vi "GeoData.vi"() -> ()   [LabVIEW 2017] (continued)
Hope\tIN\tBartholomew County\tH1\n47234\t18005\tFlat rock\tIN\tBartholomew County\tH1\n47244\t18005\tHartsville\tIN\tBartholomew County\tH1\n47226\t18005\tClifford\tIN\tBartholomew County\tH1\n47944\t18007\tFowler\tIN\tBenton County\tH1\n47917\t18007\tAmbia\tIN\tBenton County\tH1\n47975\t18007\tPine village\tIN\tBenton County\tH1\n47986\t18007\tTempleton\tIN\tBenton County\tH1\n47971\t18007\tOxford\tIN\tBenton County\tH1\n47948\t18007\tGoodland\tIN\tBenton County\tH1\n47970\t18007\tOtterbein\tIN\tBenton County\tH1\n47942\t18007\tEarl park\tIN\tBenton County\tH1\n47921\t18007\tBoswell\tIN\tBenton County\tH1\n47977\t18007\tRemington\tIN\tBenton County\tH1\n47995\t18007\tWolcott\tIN\tBenton County\tH1\n47359\t18009\tMontpelier\tIN\tBlackford County\tH1\n47348\t18009\tHartford city\tIN\tBlackford County\tH1\n47303\t18009\tMuncie\tIN\tBlackford County\tH1\n47338\t18009\tEaton\tIN\tBlackford County\tH1\n46952\t18009\tMarion\tIN\tBlackford County\tH1\n46989\t18009\tUpland\tIN\tBlackford County\tH1\n47336\t18009\tDunkirk\tIN\tBlackford County\tH1\n47369\t18009\tPennville\tIN\tBlackford County\tH1\n46147\t18011\tJamestown\tIN\tBoone County\tH1\n46268\t18011\tIndianapolis\tIN\tBoone County\tH1\n46102\t18011\tAdvance\tIN\tBoone County\tH1\n46041\t18011\tFrankfort\tIN\tBoone County\tH1\n46069\t18011\tSheridan\tIN\tBoone County\tH1\n46035\t18011\tColfax\tIN\tBoone County\tH1\n46112\t18011\tBrownsburg\tIN\tBoone County\tH1\n46052\t18011\tLebanon\tIN\tBoone County\tH1\n46077\t18011\tZionsville\tIN\tBoone County\tH1\n46278\t18011\tIndianapolis\tIN\tBoone County\tH1\n46032\t18011\tCarmel\tIN\tBoone County\tH1\n47933\t18011\tCrawfordsville\tIN\tBoone County\tH1\n47968\t18011\tNew ross\tIN\tBoone County\tH1\n46075\t18011\tWhitestown\tIN\tBoone County\tH1\n46167\t18011\tPittsboro\tIN\tBoone County\tH1\n46050\t18011\tKirklin\tIN\tBoone County\tH1\n46149\t18011\tLizton\tIN\tBoone County\tH1\n46071\t18011\tThorntown\tIN\tBoone County\tH1\n47274\t18013\tSeymour\tIN\tBrown County\tH1\n47448\t18013\tNashville\tIN\tBrown County\tH1\n47435\t18013\tHelmsburg\tIN\tBrown County\tH1\n46181\t18013\tTrafalgar\tIN\tBrown County\tH1\n47468\t18013\tUnionville\tIN\tBrown County\tH1\n47235\t18013\tFreetown\tIN\tBrown County\tH1\n47401\t18013\tBloomington\tIN\tBrown County\tH1\n46160\t18013\tMorgantown\tIN\tBrown County\tH1\n46164\t18013\tNineveh\tIN\tBrown County\tH1\n47201\t18013\tColumbus\tIN\tBrown County\tH1\n46915\t18015\tBurlington\tIN\tCarroll County\tH1\n47950\t18015\tIdaville\tIN\tCarroll County\tH1\n46929\t18015\tFlora\tIN\tCarroll County\tH1\n46917\t18015\tCamden\tIN\tCarroll County\tH1\n46913\t18015\tBringhurst\tIN\tCarroll County\tH1\n46041\t18015\tFrankfort\tIN\tCarroll County\tH1\n47960\t18015\tMonticello\tIN\tCarroll County\tH1\n46916\t18015\tBurrows\tIN\tCarroll County\tH1\n47926\t18015\tBurnettsville\tIN\tCarroll County\tH1\n46977\t18015\tRockfield\tIN\tCarroll County\tH1\n47997\t18015\tYeoman\tIN\tCarroll County\tH1\n46065\t18015\tRossville\tIN\tCarroll County\tH1\n46947\t18015\tLogansport\tIN\tCarroll County\tH1\n47905\t18015\tLafayette\tIN\tCarroll County\tH1\n47923\t18015\tBrookston\tIN\tCarroll County\tH1\n47920\t18015\tBattle ground\tIN\tCarroll County\tH1\n46920\t18015\tCutler\tIN\tCarroll County\tH1\n46923\t18015\tDelphi\tIN\tCarroll County\tH1\n46979\t18015\tRussiaville\tIN\tCarroll County\tH1\n46998\t18017\tYoung america\tIN\tCass County\tH1\n46917\t18017\tCamden\tIN\tCass County\tH1\n46926\t18017\tDenver\tIN\tCass County\tH1\n47926\t18017\tBurnettsville\tIN\tCass County\tH1\n46951\t18017\tMacy\tIN\tCass County\tH1\n46988\t18017\tTwelve mile\tIN\tCass County\tH1\n46978\t18017\tRoyal center\tIN\tCass County\tH1\n46947\t18017\tLogansport\tIN\tCass County\tH1\n46932\t18017\tGalveston\tIN\tCass County\tH1\n46950\t18017\tLucerne\tIN\tCass County\tH1\n46961\t18017\tNew waverly\tIN\tCass County\tH1\n46967\t18017\tOnward\tIN\tCass County\tH1\n46901\t18017\tKokomo\tIN\tCass County\tH1\n46970\t18017\tPeru\tIN\tCass County\tH1\n46994\t18017\tWalton\tIN\tCass County\tH1\n46942\t18017\tLake cicott\tIN\tCass County\tH1\n47119\t18019\tFloyds knobs\tIN\tClark County\tH1\n47141\t18019\tMarysville\tIN\tClark County\tH1\n47163\t18019\tOtisco\tIN\tClark County\tH1\n47243\t18019\tHanover\tIN\tClark County\tH1\n47130\t18019\tJeffersonville\tIN\tClark County\tH1\n47165\t18019\tPekin\tIN\tClark County\tH1\n47147\t18019\tNabb\tIN\tClark County\tH1\n47111\t18019\tCharlestown\tIN\tClark County\tH1\n47131\t18019\tJeffersonville\tIN\tClark County\tH1\n47172\t18019\tSellersburg\tIN\tClark County\tH1\n47190\t18019\tJeffersonville\tIN\tClark County\tH1\n47150\t18019\tNew albany\tIN\tClark County\tH1\n47126\t18019\tHenryville\tIN\tClark County\tH1\n47162\t18019\tNew washington\tIN\tClark County\tH1\n47106\t18019\tBorden\tIN\tClark County\tH1\n47143\t18019\tMemphis\tIN\tClark County\tH1\n47104\t18019\tBethlehem\tIN\tClark County\tH1\n47129\t18019\tClarksville\tIN\tClark County\tH1\n47138\t18019\tLexington\tIN\tClark County\tH1\n47177\t18019\tUnderwood\tIN\tClark County\tH1\n47802\t18021\tTerre haute\tIN\tClay County\tH1\n47840\t18021\tCenterpoint\tIN\tClay County\tH1\n47845\t18021\tCoalmont\tIN\tClay County\tH1\n47853\t18021\tHarmony\tIN\tClay County\tH1\n47857\t18021\tKnightsville\tIN\tClay County\tH1\n47868\t18021\tPoland\tIN\tClay County\tH1\n47427\t18021\tCoal city\tIN\tClay County\tH1\n47858\t18021\tLewis\tIN\tClay County\tH1\n47841\t18021\tClay city\tIN\tClay County\tH1\n47881\t18021\tStaunton\tIN\tClay County\tH1\n47834\t18021\tBrazil\tIN\tClay County\tH1\n47879\t18021\tShelburn\tIN\tClay County\tH1\n47803\t18021\tTerre haute\tIN\tClay County\tH1\n47438\t18021\tJasonville\tIN\tClay County\tH1\n47874\t18021\tRosedale\tIN\tClay County\tH1\n47846\t18021\tCory\tIN\tClay County\tH1\n47837\t18021\tCarbon\tIN\tClay County\tH1\n47833\t18021\tBowling green\tIN\tClay County\tH1\n46039\t18023\tForest\tIN\tClinton County\tH1\n46041\t18023\tFrankfort\tIN\tClinton County\tH1\n46069\t18023\tSheridan\tIN\tClinton County\tH1\n46035\t18023\tColfax\tIN\tClinton County\tH1\n46067\t18023\tSedalia\tIN\tClinton County\tH1\n46065\t18023\tRossville\tIN\tClinton County\tH1\n46057\t18023\tMichigantown\tIN\tClinton County\tH1\n46049\t18023\tKempton\tIN\tClinton County\tH1\n46058\t18023\tMulberry\tIN\tClinton County\tH1\n46050\t18023\tKirklin\tIN\tClinton County\tH1\n46979\t18023\tRussiaville\tIN\tClinton County\tH1\n46071\t18023\tThorntown\tIN\tClinton County\tH1\n47930\t18023\tClarks hill\tIN\tClinton County\tH1\n47175\t18025\tTaswell\tIN\tCrawford County\tH1\n47576\t18025\tSaint croix\tIN\tCrawford County\tH1\n47116\t18025\tEckerty\tIN\tCrawford County\tH1\n47123\t18025\tGrantsburg\tIN\tCrawford County\tH1\n47174\t18025\tSulphur\tIN\tCrawford County\tH1\n47145\t18025\tMilltown\tIN\tCrawford County\tH1\n47140\t18025\tMarengo\tIN\tCrawford County\tH1\n47112\t18025\tCorydon\tIN\tCrawford County\tH1\n47137\t18025\tLeavenworth\tIN\tCrawford County\tH1\n47118\t18025\tEnglish\tIN\tCrawford County\tH1\n47513\t18025\tBirdseye\tIN\tCrawford County\tH1\n47553\t18027\tLoogootee\tIN\tDaviess County\tH1\n47562\t18027\tOdon\tIN\tDaviess County\tH1\n47529\t18027\tElnora\tIN\tDaviess County\tH1\n47501\t18027\tWashington\tIN\tDaviess County\tH1\n47519\t18027\tCannelburg\tIN\tDaviess County\tH1\n47568\t18027\tPlainville\tIN\tDaviess County\tH1\n47558\t18027\tMontgomery\tIN\tDaviess County\tH1\n47449\t18027\tNewberry\tIN\tDaviess County\tH1\n47001\t18029\tAurora\tIN\tDearborn County\tH1\n47018\t18029\tDillsboro\tIN\tDearborn County\tH1\n47060\t18029\tWest harrison\tIN\tDearborn County\tH1\n47012\t18029\tBrookville\tIN\tDearborn County\tH1\n47032\t18029\tMoores hill\tIN\tDearborn County\tH1\n47025\t18029\tLawrenceburg\tIN\tDearborn County\tH1\n47022\t18029\tGuilford\tIN\tDearborn County\tH1\n47041\t18029\tSunman\tIN\tDearborn County\tH1\n47031\t18029\tMilan\tIN\tDearborn County\tH1\n46156\t18031\tMilroy\tIN\tDecatur County\tH1\n47240\t18031\tGreensburg\tIN\tDecatur County\tH1\n47225\t18031\tClarksburg\tIN\tDecatur County\tH1\n47263\t18031\tNew point\tIN\tDecatur County\tH1\n46173\t18031\tRushville\tIN\tDecatur County\tH1\n47272\t18031\tSaint paul\tIN\tDecatur County\tH1\n47283\t18031\tWestport\tIN\tDecatur County\tH1\n47006\t18031\tBatesville\tIN\tDecatur County\tH1\n47246\t18031\tHope\tIN\tDecatur County\tH1\n47244\t18031\tHartsville\tIN\tDecatur County\tH1\n46747\t18033\tHudson\tIN\tDeKalb County\tH1\n46742\t18033\tHamilton\tIN\tDeKalb County\tH1\n46730\t18033\tCorunna\tIN\tDeKalb County\tH1\n46748\t18033\tHuntertown\tIN\tDeKalb County\tH1\n46743\t18033\tHarlan\tIN\tDeKalb County\tH1\n46755\t18033\tKendallville\tIN\tDeKalb County\tH1\n46793\t18033\tWaterloo\tIN\tDeKalb County\tH1\n46706\t18033\tAuburn\tIN\tDeKalb County\tH1\n46710\t18033\tAvilla\tIN\tDeKalb County\tH1\n46785\t18033\tSaint joe\tIN\tDeKalb County\tH1\n46738\t18033\tGarrett\tIN\tDeKalb County\tH1\n46763\t18033\tLaotto\tIN\tDeKalb County\tH1\n46721\t18033\tButler\tIN\tDeKalb County\tH1\n46705\t18033\tAshley\tIN\tDeKalb County\tH1\n46788\t18033\tSpencerville\tIN\tDeKalb County\tH1\n46012\t18035\tAnderson\tIN\tDelaware County\tH1\n47306\t18035\tMuncie\tIN\tDelaware County\tH1\n47302\t18035\tMuncie\tIN\tDelaware County\tH1\n47320\t18035\tAlbany\tIN\tDelaware County\tH1\n47386\t18035\tSpringport\tIN\tDelaware County\tH1\n47303\t18035\tMuncie\tIN\tDelaware County\tH1\n47338\t18035\tEaton\tIN\tDelaware County\tH1\n47342\t18035\tGaston\tIN\tDelaware County\tH1\n47304\t18035\tMuncie\tIN\tDelaware County\tH1\n47396\t18035\tYorktown\tIN\tDelaware County\tH1\n47308\t18035\tMuncie\tIN\tDelaware County\tH1\n47383\t18035\tSelma\tIN\tDelaware County\tH1\n46001\t18035\tAlexandria\tIN\tDelaware County\tH1\n47336\t18035\tDunkirk\tIN\tDelaware County\tH1\n47307\t18035\tMuncie\tIN\tDelaware County\tH1\n47367\t18035\tOakville\tIN\tDelaware County\tH1\n46017\t18035\tAnderson\tIN\tDelaware County\tH1\n46070\t18035\tSummitville\tIN\tDelaware County\tH1\n47356\t18035\tMiddletown\tIN\tDelaware County\tH1\n47334\t18035\tDaleville\tIN\tDelaware County\tH1\n47368\t18035\tParker city\tIN\tDelaware County\tH1\n47354\t18035\tLosantville\tIN\tDelaware County\tH1\n47305\t18035\tMuncie\tIN\tDelaware County\tH1\n47523\t18037\tDale\tIN\tDubois County\tH1\n47542\t18037\tHuntingburg\tIN\tDubois County\tH1\n47547\t18037\tJasper\tIN\tDubois County\tH1\n47575\t18037\tSaint anthony\tIN\tDubois County\tH1\n47527\t18037\tDubois\tIN\tDubois County\tH1\n47564\t18037\tOtwell\tIN\tDubois County\tH1\n47580\t18037\tSchnellville\tIN\tDubois County\tH1\n47541\t18037\tHolland\tIN\tDubois County\tH1\n47590\t18037\tVelpen\tIN\tDubois County\tH1\n47546\t18037\tJasper\tIN\tDubois County\tH1\n47432\t18037\tFrench lick\tIN\tDubois County\tH1\n47521\t18037\tCelestine\tIN\tDubois County\tH1\n47545\t18037\tIreland\tIN\tDubois County\tH1\n47532\t18037\tFerdinand\tIN\tDubois County\tH1\n47513\t18037\tBirdseye\tIN\tDubois County\tH1\n46514\t18039\tElkhart\tIN\tElkhart County\tH1\n46516\t18039\tElkhart\tIN\tElkhart County\tH1\n46567\t18039\tSyracuse\tIN\tElkhart County\tH1\n46542\t18039\tMilford\tIN\tElkhart County\tH1\n46561\t18039\tOsceola\tIN\tElkhart County\tH1\n46565\t18039\tShipshewana\tIN\tElkhart County\tH1\n46550\t18039\tNappanee\tIN\tElkhart County\tH1\n46527\t18039\tGoshen\tIN\tElkhart County\tH1\n46553\t18039\tNew paris\tIN\tElkhart County\tH1\n46517\t18039\tElkhart\tIN\tElkhart County\tH1\n46530\t18039\tGranger\tIN\tElkhart County\tH1\n46515\t18039\tElkhart\tIN\tElkhart County\tH1\n46573\t18039\tWakarusa\tIN\tElkhart County\tH1\n46526\t18039\tGoshen\tIN\tElkhart County\tH1\n46540\t18039\tMiddlebury\tIN\tElkhart County\tH1\n46528\t18039\tGoshen\tIN\tElkhart County\tH1\n46543\t18039\tMillersburg\tIN\tElkhart County\tH1\n46767\t18039\tLigonier\tIN\tElkhart County\tH1\n46507\t18039\tBristol\tIN\tElkhart County\tH1\n47331\t18041\tConnersville\tIN\tFayette County\tH1\n46127\t18041\tFalmouth\tIN\tFayette County\tH1\n47327\t18041\tCambridge city\tIN\tFayette County\tH1\n47352\t18041\tLewisville\tIN\tFayette County\tH1\n46173\t18041\tRushville\tIN\tFayette County\tH1\n46133\t18041\tGlenwood\tIN\tFayette County\tH1\n47024\t18041\tLaurel\tIN\tFayette County\tH1\n47325\t18041\tBrownsville\tIN\tFayette County\tH1\n47357\t18041\tMilton\tIN\tFayette County\tH1\n47322\t18041\tBentonville\tIN\tFayette County\tH1\n47164\t18043\tPalmyra\tIN\tFloyd County\tH1\n47119\t18043\tFloyds knobs\tIN\tFloyd County\tH1\n47165\t18043\tPekin\tIN\tFloyd County\tH1\n47172\t18043\tSellersburg\tIN\tFloyd County\tH1\n47150\t18043\tNew albany\tIN\tFloyd County\tH1\n47117\t18043\tElizabeth\tIN\tFloyd County\tH1\n47136\t18043\tLanesville\tIN\tFloyd County\tH1\n47106\t18043\tBorden\tIN\tFloyd County\tH1\n47122\t18043\tGeorgetown\tIN\tFloyd County\tH1\n47124\t18043\tGreenville\tIN\tFloyd County\tH1\n47151\t18043\tNew albany\tIN\tFloyd County\tH1\n47146\t18043\tMount saint francis\tIN\tFloyd County\tH1\n47958\t18045\tMellott\tIN\tFountain County\tH1\n47990\t18045\tWaynetown\tIN\tFountain County\tH1\n47992\t18045\tWestpoint\tIN\tFountain County\tH1\n47952\t18045\tKingman\tIN\tFountain County\tH1\n47933\t18045\tCrawfordsville\tIN\tFountain County\tH1\n47932\t18045\tCovington\tIN\tFountain County\tH1\n47987\t18045\tVeedersburg\tIN\tFountain County\tH1\n47994\t18045\tWingate\tIN\tFountain County\tH1\n47949\t18045\tHillsboro\tIN\tFountain County\tH1\n47969\t18045\tNewtown\tIN\tFountain County\tH1\n47918\t18045\tAttica\tIN\tFountain County\tH1\n47060\t18047\tWest harrison\tIN\tFranklin County\tH1\n47240\t18047\tGreensburg\tIN\tFranklin County\tH1\n47331\t18047\tConnersville\tIN\tFranklin County\tH1\n47036\t18047\tOldenburg\tIN\tFranklin County\tH1\n47010\t18047\tBath\tIN\tFranklin County\tH1\n47012\t18047\tBrookville\tIN\tFranklin County\tH1\n46173\t18047\tRushville\tIN\tFranklin County\tH1\n47353\t18047\tLiberty\tIN\tFranklin County\tH1\n47006\t18047\tBatesville\tIN\tFranklin County\tH1\n47030\t18047\tMetamora\tIN\tFranklin County\tH1\n47003\t18047\tWest college corner\tIN\tFranklin County\tH1\n47024\t18047\tLaurel\tIN\tFranklin County\tH1\n47041\t18047\tSunman\tIN\tFranklin County\tH1\n47016\t18047\tCedar grove\tIN\tFranklin County\tH1\n47035\t18047\tNew trenton\tIN\tFranklin County\tH1\n46910\t18049\tAkron\tIN\tFulton County\tH1\n46945\t18049\tLeiters ford\tIN\tFulton County\tH1\n46570\t18049\tTippecanoe\tIN\tFulton County\tH1\n46912\t18049\tAthens\tIN\tFulton County\tH1\n46951\t18049\tMacy\tIN\tFulton County\tH1\n46985\t18049\tStar city\tIN\tFulton County\tH1\n46978\t18049\tRoyal center\tIN\tFulton County\tH1\n46922\t18049\tDelong\tIN\tFulton County\tH1\n46539\t18049\tMentone\tIN\tFulton County\tH1\n46982\t18049\tSilver lake\tIN\tFulton County\tH1\n46960\t18049\tMonterey\tIN\tFulton County\tH1\n46931\t18049\tFulton\tIN\tFulton County\tH1\n46501\t18049\tArgos\tIN\tFulton County\tH1\n46950\t18049\tLucerne\tIN\tFulton County\tH1\n46511\t18049\tCulver\tIN\tFulton County\tH1\n46939\t18049\tKewanna\tIN\tFulton County\tH1\n46975\t18049\tRochester\tIN\tFulton County\tH1\n47633\t18051\tPoseyville\tIN\tGibson County\tH1\n47616\t18051\tGriffin\tIN\tGibson County\tH1\n47660\t18051\tOakland city\tIN\tGibson County\tH1\n47613\t18051\tElberfeld\tIN\tGibson County\tH1\n47665\t18051\tOwensville\tIN\tGibson County\tH1\n47648\t18051\tFort branch\tIN\tGibson County\tH1\n47666\t18051\tPatoka\tIN\tGibson County\tH1\n47725\t18051\tEvansville\tIN\tGibson County\tH1\n47654\t18051\tMackey\tIN\tGibson County\tH1\n47683\t18051\tSomerville\tIN\tGibson County\tH1\n47612\t18051\tCynthiana\tIN\tGibson County\tH1\n47639\t18051\tHaubstadt\tIN\tGibson County\tH1\n47647\t18051\tBuckskin\tIN\tGibson County\tH1\n47619\t18051\tLynnville\tIN\tGibson County\tH1\n47670\t18051\tPrinceton\tIN\tGibson County\tH1\n47640\t18051\tHazleton\tIN\tGibson County\tH1\n47649\t18051\tFrancisco\tIN\tGibson County\tH1\n46933\t18053\tGas city\tIN\tGrant County\tH1\n46930\t18053\tFowlerton\tIN\tGrant County\tH1\n46986\t18053\tSwayzee\tIN\tGrant County\tH1\n46919\t18053\tConverse\tIN\tGrant County\tH1\n46991\t18053\tVan buren\tIN\tGrant County\tH1\n46987\t18053\tSweetser\tIN\tGrant County\tH1\n47348\t18053\tHartford city\tIN\tGrant County\tH1\n47342\t18053\tGaston\tIN\tGrant County\tH1\n46957\t18053\tMatthews\tIN\tGrant County\tH1\n46952\t18053\tMarion\tIN\tGrant County\tH1\n46953\t18053\tMarion\tIN\tGrant County\tH1\n46989\t18053\tUpland\tIN\tGrant County\tH1\n46928\t18053\tFairmount\tIN\tGrant County\tH1\n46036\t18053\tElwood\tIN\tGrant County\tH1\n46938\t18053\tJonesboro\tIN\tGrant County\tH1\n46940\t18053\tLa fontaine\tIN\tGrant County\tH1\n46070\t18053\tSummitville\tIN\tGrant County\tH1\n47441\t18055\tLinton\tIN\tGreene County\tH1\n47424\t18055\tBloomfield\tIN\tGreene County\tH1\n47465\t18055\tSwitz city\tIN\tGreene County\tH1\n47445\t18055\tMidland\tIN\tGreene County\tH1\n47471\t18055\tWorthington\tIN\tGreene County\tH1\n47562\t18055\tOdon\tIN\tGreene County\tH1\n47453\t18055\tOwensburg\tIN\tGreene County\tH1\n47529\t18055\tElnora\tIN\tGreene County\tH1\n47459\t18055\tSolsberry\tIN\tGreene County\tH1\n47848\t18055\tDugger\tIN\tGreene County\tH1\n47403\t18055\tBloomington\tIN\tGreene County\tH1\n47462\t18055\tSpringville\tIN\tGreene County\tH1\n47460\t18055\tSpencer\tIN\tGreene County\tH1\n47438\t18055\tJasonville\tIN\tGreene County\tH1\n47838\t18055\tCarlisle\tIN\tGreene County\tH1\n47443\t18055\tLyons\tIN\tGreene County\tH1\n47578\t18055\tSandborn\tIN\tGreene County\tH1\n47457\t18055\tScotland\tIN\tGreene County\tH1\n47449\t18055\tNewberry\tIN\tGreene County\tH1\n46268\t18057\tIndianapolis\tIN\tHamilton County\tH1\n46040\t18057\tFortville\tIN\tHamilton County\tH1\n46060\t18057\tNoblesville\tIN\tHamilton County\tH1\n46031\t18057\tAtlanta\tIN\tHamilton County\tH1\n46082\t18057\tCarmel\tIN\tHamilton County\tH1\n46260\t18057\tIndianapolis\tIN\tHamilton County\tH1\n46280\t18057\tIndianapolis\tIN\tHamilton County\tH1\n46290\t18057\tIndianapolis\tIN\tHamilton County\tH1\n46250\t18057\tIndianapolis\tIN\tHamilton County\tH1\n46037\t18057\tFishers\tIN\tHamilton County\tH1\n46033\t18057\tCarmel\tIN\tHamilton County\tH1\n46062\t18057\tNoblesville\tIN\tHamilton County\tH1\n46034\t18057\tCicero\tIN\tHamilton County\tH1\n46069\t18057\tSheridan\tIN\tHamilton County\tH1\n46256\t18057\tIndianapolis\tIN\tHamilton County\tH1\n46030\t18057\tArcadia\tIN\tHamilton County\tH1\n46055\t18057\tMccordsville\tIN\tHamilton County\tH1\n46077\t18057\tZionsville\tIN\tHamilton County\tH1\n46236\t18057\tIndianapolis\tIN\tHamilton County\tH1\n46032\t18057\tCarmel\tIN\tHamilton County\tH1\n46061\t18057\tNoblesville\tIN\tHamilton County\tH1\n46240\t18057\tIndianapolis\tIN\tHamilton County\tH1\n46011\t18057\tAnderson\tIN\tHamilton County\tH1\n46038\t18057\tFishers\tIN\tHamilton County\tH1\n46036\t18057\tElwood\tIN\tHamilton County\tH1\n46064\t18057\tPendleton\tIN\tHamilton County\tH1\n46049\t18057\tKempton\tIN\tHamilton County\tH1\n46074\t18057\tWestfield\tIN\tHamilton County\tH1\n46072\t18057\tTipton\tIN\tHamilton County\tH1\n46050\t18057\tKirklin\tIN\tHamilton County\tH1\n46229\t18059\tIndianapolis\tIN\tHancock County\tH1\n46040\t18059\tFortville\tIN\tHancock County\tH1\n46056\t18059\tMarkleville\tIN\tHancock County\tH1\n46148\t18059\tKnightstown\tIN\tHancock County\tH1\n46115\t18059\tCarthage\tIN\tHancock County\tH1\n46055\t18059\tMccordsville\tIN\tHancock County\tH1\n46130\t18059\tFountaintown\tIN\tHancock County\tH1\n46163\t18059\tNew palestine\tIN\tHancock County\tH1\n46236\t18059\tIndianapolis\tIN\tHancock County\tH1\n46154\t18059\tMaxwell\tIN\tHancock County\tH1\n46140\t18059\tGreenfield\tIN\tHancock County\tH1\n46161\t18059\tMorristown\tIN\tHancock County\tH1\n46064\t18059\tPendleton\tIN\tHancock County\tH1\n47384\t18059\tShirley\tIN\tHancock County\tH1\n46117\t18059\tCharlottesville\tIN\tHancock County\tH1\n46186\t18059\tWilkinson\tIN\tHancock County\tH1\n46239\t18059\tIndianapolis\tIN\tHancock County\tH1\n47164\t18061\tPalmyra\tIN\tHarrison County\tH1\n47142\t18061\tMauckport\tIN\tHarrison County\tH1\n47107\t18061\tBradford\tIN\tHarrison County\tH1\n47125\t18061\tHardinsburg\tIN\tHarrison County\tH1\n47160\t18061\tNew middletown\tIN\tHarrison County\tH1\n47114\t18061\tCrandall\tIN\tHarrison County\tH1\n47115\t18061\tDepauw\tIN\tHarrison County\tH1\n47112\t18061\tCorydon\tIN\tHarrison County\tH1\n47117\t18061\tElizabeth\tIN\tHarrison County\tH1\n47136\t18061\tLanesville\tIN\tHarrison County\tH1\n47110\t18061\tCentral\tIN\tHarrison County\tH1\n47137\t18061\tLeavenworth\tIN\tHarrison County\tH1\n47166\t18061\tRamsey\tIN\tHarrison County\tH1\n47122\t18061\tGeorgetown\tIN\tHarrison County\tH1\n47135\t18061\tLaconia\tIN\tHarrison County\tH1\n47161\t18061\tNew salisbury\tIN\tHarrison County\tH1\n47124\t18061\tGreenville\tIN\tHarrison County\tH1\n47120\t18061\tFredericksburg\tIN\tHarrison County\tH1\n46158\t18063\tMooresville\tIN\tHendricks County\tH1\n46147\t18063\tJamestown\tIN\tHendricks County\tH1\n46168\t18063\tPlainfield\tIN\tHendricks County\tH1\n46112\t18063\tBrownsburg\tIN\tHendricks County\tH1\n46234\t18063\tIndianapolis\tIN\tHendricks County\tH1\n46231\t18063\tIndianapolis\tIN\tHendricks County\tH1\n46052\t18063\tLebanon\tIN\tHendricks County\tH1\n46123\t18063\tAvon\tIN\tHendricks County\tH1\n46077\t18063\tZionsville\tIN\tHendricks County\tH1\n46122\t18063\tDanville\tIN\tHendricks County\tH1\n46157\t18063\tMonrovia\tIN\tHendricks County\tH1\n46113\t18063\tCamby\tIN\tHendricks County\tH1\n46278\t18063\tIndianapolis\tIN\tHendricks County\tH1\n47968\t18063\tNew ross\tIN\tHendricks County\tH1\n46180\t18063\tStilesville\tIN\tHendricks County\tH1\n46167\t18063\tPittsboro\tIN\tHendricks County\tH1\n46165\t18063\tNorth salem\tIN\tHendricks County\tH1\n46118\t18063\tClayton\tIN\tHendricks County\tH1\n46149\t18063\tLizton\tIN\tHendricks County\tH1\n46121\t18063\tCoatesville\tIN\tHendricks County\tH1\n46239\t18063\tIndianapolis\tIN\tHendricks County\tH1\n46103\t18063\tAmo\tIN\tHendricks County\tH1\n46056\t18065\tMarkleville\tIN\tHenry County\tH1\n47346\t18065\tHagerstown\tIN\tHenry County\tH1\n46148\t18065\tKnightstown\tIN\tHenry County\tH1\n47302\t18065\tMuncie\tIN\tHenry County\tH1\n47386\t18065\tSpringport\tIN\tHenry County\tH1\n47351\t18065\tKennard\tIN\tHenry County\tH1\n47387\t18065\tStraughn\tIN\tHenry County\tH1\n47344\t18065\tGreensboro\tIN\tHenry County\tH1\n47327\t18065\tCambridge city\tIN\tHenry County\tH1\n47385\t18065\tSpiceland\tIN\tHenry County\tH1\n47352\t18065\tLewisville\tIN\tHenry County\tH1\n47366\t18065\tNew lisbon\tIN\tHenry County\tH1\n47362\t18065\tNew castle\tIN\tHenry County\tH1\n47337\t18065\tDunreith\tIN\tHenry County\tH1\n47361\t18065\tMount summit\tIN\tHenry County\tH1\n47388\t18065\tSulphur springs\tIN\tHenry County\tH1\n47356\t18065\tMiddletown\tIN\tHenry County\tH1\n47334\t18065\tDaleville\tIN\tHenry County\tH1\n47384\t18065\tShirley\tIN\tHenry County\tH1\n47360\t18065\tMooreland\tIN\tHenry County\tH1\n47354\t18065\tLosantville\tIN\tHenry County\tH1\n46117\t18065\tCharlottesville\tIN\tHenry County\tH1\n46186\t18065\tWilkinson\tIN\tHenry County\tH1\n46902\t18067\tKokomo\tIN\tHoward County\tH1\n46919\t18067\tConverse\tIN\tHoward County\tH1\n46039\t18067\tForest\tIN\tHoward County\tH1\n46076\t18067\tWindfall\tIN\tHoward County\tH1\n46929\t18067\tFlora\tIN\tHoward County\tH1\n46041\t18067\tFrankfort\tIN\tHoward County\tH1\n46936\t18067\tGreentown\tIN\tHoward County\tH1\n46995\t18067\tWest middleton\tIN\tHoward County\tH1\n46903\t18067\tKokomo\tIN\tHoward County\tH1\n46937\t18067\tHemlock\tIN\tHoward County\tH1\n46068\t18067\tSharpsville\tIN\tHoward County\tH1\n46904\t18067\tKokomo\tIN\tHoward County\tH1\n46928\t18067\tFairmount\tIN\tHoward County\tH1\n46932\t18067\tGalveston\tIN\tHoward County\tH1\n46965\t18067\tOakford\tIN\tHoward County\tH1\n46901\t18067\tKokomo\tIN\tHoward County\tH1\n46979\t18067\tRussiaville\tIN\tHoward County\tH1\n46725\t18069\tColumbia city\tIN\tHuntington County\tH1\n46991\t18069\tVan buren\tIN\tHuntington County\tH1\n46783\t18069\tRoanoke\tIN\tHuntington County\tH1\n46713\t18069\tBippus\tIN\tHuntington County\tH1\n46750\t18069\tHuntington\tIN\tHuntington County\tH1\n46770\t18069\tMarkle\tIN\tHuntington County\tH1\n46766\t18069\tLiberty center\tIN\tHuntington County\tH1\n46792\t18069\tWarren\tIN\tHuntington County\tH1\n46952\t18069\tMarion\tIN\tHuntington County\tH1\n46787\t18069\tSouth whitley\tIN\tHuntington County\tH1\n46940\t18069\tLa fontaine\tIN\tHuntington County\tH1\n46702\t18069\tAndrews\tIN\tHuntington County\tH1\n47229\t18071\tCrothersville\tIN\tJackson County\tH1\n47274\t18071\tSeymour\tIN\tJackson County\tH1\n47281\t18071\tVallonia\tIN\tJackson County\tH1\n47102\t18071\tAustin\tIN\tJackson County\tH1\n47235\t18071\tFreetown\tIN\tJackson County\tH1\n47228\t18071\tCortland\tIN\tJackson County\tH1\n47220\t18071\tBrownstown\tIN\tJackson County\tH1\n47260\t18071\tMedora\tIN\tJackson County\tH1\n47264\t18071\tNorman\tIN\tJackson County\tH1\n47201\t18071\tColumbus\tIN\tJackson County\tH1\n46380\t18073\tTefft\tIN\tJasper County\tH1\n46310\t18073\tDemotte\tIN\tJasper County\tH1\n47978\t18073\tRensselaer\tIN\tJasper County\tH1\n47959\t18073\tMonon\tIN\tJasper County\tH1\n46341\t18073\tHebron\tIN\tJasper County\tH1\n46374\t18073\tSan pierre\tIN\tJasper County\tH1\n47948\t18073\tGoodland\tIN\tJasper County\tH1\n47946\t18073\tFrancesville\tIN\tJasper County\tH1\n47922\t18073\tBrook\tIN\tJasper County\tH1\n47957\t18073\tMedaryville\tIN\tJasper County\tH1\n46392\t18073\tWheatfield\tIN\tJasper County\tH1\n47977\t18073\tRemington\tIN\tJasper County\tH1\n47943\t18073\tFair oaks\tIN\tJasper County\tH1\n47995\t18073\tWolcott\tIN\tJasper County\tH1\n47390\t18075\tUnion city\tIN\tJay County\tH1\n47359\t18075\tMontpelier\tIN\tJay County\tH1\n47373\t18075\tRedkey\tIN\tJay County\tH1\n47320\t18075\tAlbany\tIN\tJay County\tH1\n47380\t18075\tRidgeville\tIN\tJay County\tH1\n47326\t18075\tBryant\tIN\tJay County\tH1\n46740\t18075\tGeneva\tIN\tJay County\tH1\n47336\t18075\tDunkirk\tIN\tJay County\tH1\n47371\t18075\tPortland\tIN\tJay County\tH1\n47381\t18075\tSalamonia\tIN\tJay County\tH1\n47369\t18075\tPennville\tIN\tJay County\tH1\n47224\t18077\tCanaan\tIN\tJefferson County\tH1\n47043\t18077\tVevay\tIN\tJefferson County\tH1\n47011\t18077\tBennington\tIN\tJefferson County\tH1\n47243\t18077\tHanover\tIN\tJefferson County\tH1\n47147\t18077\tNabb\tIN\tJefferson County\tH1\n47170\t18077\tScottsburg\tIN\tJefferson County\tH1\n47231\t18077\tDupont\tIN\tJefferson County\tH1\n47250\t18077\tMadison\tIN\tJefferson County\tH1\n47138\t18077\tLexington\tIN\tJefferson County\tH1\n47230\t18077\tDeputy\tIN\tJefferson County\tH1\n47270\t18077\tParis crossing\tIN\tJefferson County\tH1\n47227\t18077\tCommiskey\tIN\tJefferson County\tH1\n47229\t18079\tCrothersville\tIN\tJennings County\tH1\n47274\t18079\tSeymour\tIN\tJennings County\tH1\n47273\t18079\tScipio\tIN\tJennings County\tH1\n47245\t18079\tHayden\tIN\tJennings County\tH1\n47232\t18079\tElizabethtown\tIN\tJennings County\tH1\n47231\t18079\tDupont\tIN\tJennings County\tH1\n47283\t18079\tWestport\tIN\tJennings County\tH1\n47282\t18079\tVernon\tIN\tJennings County\tH1\n47223\t18079\tButlerville\tIN\tJennings County\tH1\n47037\t18079\tOsgood\tIN\tJennings County\tH1\n47265\t18079\tNorth vernon\tIN\tJennings County\tH1\n47230\t18079\tDeputy\tIN\tJennings County\tH1\n47270\t18079\tParis crossing\tIN\tJennings County\tH1\n47227\t18079\tCommiskey\tIN\tJennings County\tH1\n46106\t18081\tBargersville\tIN\tJohnson County\tH1\n46143\t18081\tGreenwood\tIN\tJohnson County\tH1\n46142\t18081\tGreenwood\tIN\tJohnson County\tH1\n46162\t18081\tNeedham\tIN\tJohnson County\tH1\n46181\t18081\tTrafalgar\tIN\tJohnson County\tH1\n46110\t18081\tBoggstown\tIN\tJohnson County\tH1\n46184\t18081\tWhiteland\tIN\tJohnson County\tH1\n46160\t18081\tMorgantown\tIN\tJohnson County\tH1\n46164\t18081\tNineveh\tIN\tJohnson County\tH1\n46131\t18081\tFranklin\tIN\tJohnson County\tH1\n46151\t18081\tMartinsville\tIN\tJohnson County\tH1\n46124\t18081\tEdinburgh\tIN\tJohnson County\tH1\n46259\t18081\tIndianapolis\tIN\tJohnson County\tH1\n47596\t18083\tWestphalia\tIN\tKnox County\tH1\n47516\t18083\tBruceville\tIN\tKnox County\tH1\n47573\t18083\tRagsdale\tIN\tKnox County\tH1\n47535\t18083\tFreelandville\tIN\tKnox County\tH1\n47591\t18083\tVincennes\tIN\tKnox County\tH1\n47597\t18083\tWheatland\tIN\tKnox County\tH1\n47528\t18083\tEdwardsport\tIN\tKnox County\tH1\n47561\t18083\tOaktown\tIN\tKnox County\tH1\n47524\t18083\tDecker\tIN\tKnox County\tH1\n47838\t18083\tCarlisle\tIN\tKnox County\tH1\n47578\t18083\tSandborn\tIN\tKnox County\tH1\n47512\t18083\tBicknell\tIN\tKnox County\tH1\n47557\t18083\tMonroe city\tIN\tKnox County\tH1\n46504\t18085\tBourbon\tIN\tKosciusko County\tH1\n46567\t18085\tSyracuse\tIN\tKosciusko County\tH1\n46524\t18085\tEtna green\tIN\tKosciusko County\tH1\n46910\t18085\tAkron\tIN\tKosciusko County\tH1\n46732\t18085\tCromwell\tIN\tKosciusko County\tH1\n46542\t18085\tMilford\tIN\tKosciusko County\tH1\n46508\t18085\tBurket\tIN\tKosciusko County\tH1\n46550\t18085\tNappanee\tIN\tKosciusko County\tH1\n46582\t18085\tWarsaw\tIN\tKosciusko County\tH1\n46580\t18085\tWarsaw\tIN\tKosciusko County\tH1\n46506\t18085\tBremen\tIN\tKosciusko County\tH1\n46555\t18085\tNorth webster\tIN\tKosciusko County\tH1\n46510\t18085\tClaypool\tIN\tKosciusko County\tH1\n46539\t18085\tMentone\tIN\tKosciusko County\tH1\n46581\t18085\tWarsaw\tIN\tKosciusko County\tH1\n46562\t18085\tPierceton\tIN\tKosciusko County\tH1\n46982\t18085\tSilver lake\tIN\tKosciusko County\tH1\n46962\t18085\tNorth manchester\tIN\tKosciusko County\tH1\n46538\t18085\tLeesburg\tIN\tKosciusko County\tH1\n46590\t18085\tWinona lake\tIN\tKosciusko County\tH1\n46787\t18085\tSouth whitley\tIN\tKosciusko County\tH1\n46767\t18085\tLigonier\tIN\tKosciusko County\tH1\n46975\t18085\tRochester\tIN\tKosciusko County\tH1\n46502\t18085\tAtwood\tIN\tKosciusko County\tH1\n46746\t18087\tHowe\tIN\tLaGrange County\tH1\n46565\t18087\tShipshewana\tIN\tLaGrange County\tH1\n46747\t18087\tHudson\tIN\tLaGrange County\tH1\n46786\t18087\tSouth milford\tIN\tLaGrange County\tH1\n46776\t18087\tOrland\tIN\tLaGrange County\tH1\n46571\t18087\tTopeka\tIN\tLaGrange County\tH1\n46784\t18087\tRome city\tIN\tLaGrange County\tH1\n46789\t18087\tStroh\tIN\tLaGrange County\tH1\n46540\t18087\tMiddlebury\tIN\tLaGrange County\tH1\n46528\t18087\tGoshen\tIN\tLaGrange County\tH1\n46543\t18087\tMillersburg\tIN\tLaGrange County\tH1\n46767\t18087\tLigonier\tIN\tLaGrange County\tH1\n46761\t18087\tLagrange\tIN\tLaGrange County\tH1\n46795\t18087\tWolcottville\tIN\tLaGrange County\tH1\n46771\t18087\tMongo\tIN\tLaGrange County\tH1\n46311\t18089\tDyer\tIN\tLake County\tH1\n46408\t18089\tGary\tIN\tLake County\tH1\n46411\t18089\tMerrillville\tIN\tLake County\tH1\n46355\t18089\tLeroy\tIN\tLake County\tH1\n46323\t18089\tHammond\tIN\tLake County\tH1\n46356\t18089\tLowell\tIN\tLake County\tH1\n46373\t18089\tSaint john\tIN\tLake County\tH1\n46375\t18089\tSchererville\tIN\tLake County\tH1\n46376\t18089\tSchneider\tIN\tLake County\tH1\n46320\t18089\tHammond\tIN\tLake County\tH1\n46321\t18089\tMunster\tIN\tLake County\tH1\n46322\t18089\tHighland\tIN\tLake County\tH1\n46403\t18089\tGary\tIN\tLake County\tH1\n46410\t18089\tMerrillville\tIN\tLake County\tH1\n46404\t18089\tGary\tIN\tLake County\tH1\n46409\t18089\tGary\tIN\tLake County\tH1\n46341\t18089\tHebron\tIN\tLake County\tH1\n46303\t18089\tCedar lake\tIN\tLake County\tH1\n46307\t18089\tCrown point\tIN\tLake County\tH1\n46324\t18089\tHammond\tIN\tLake County\tH1\n46327\t18089\tHammond\tIN\tLake County\tH1\n46383\t18089\tValparaiso\tIN\tLake County\tH1\n46394\t18089\tWhiting\tIN\tLake County\tH1\n46407\t18089\tGary\tIN\tLake County\tH1\n46312\t18089\tEast chicago\tIN\tLake County\tH1\n46368\t18089\tPortage\tIN\tLake County\tH1\n46402\t18089\tGary\tIN\tLake County\tH1\n46405\t18089\tLake station\tIN\tLake County\tH1\n46401\t18089\tGary\tIN\tLake County\tH1\n46308\t18089\tCrown point\tIN\tLake County\tH1\n46377\t18089\tShelby\tIN\tLake County\tH1\n46319\t18089\tGriffith\tIN\tLake County\tH1\n46342\t18089\tHobart\tIN\tLake County\tH1\n46406\t18089\tGary\tIN\tLake County\tH1\n46391\t18091\tWestville\tIN\tLaPorte County\tH1\n46552\t18091\tNew carlisle\tIN\tLaPorte County\tH1\n46346\t18091\tKingsford heights\tIN\tLaPorte County\tH1\n46345\t18091\tKingsbury\tIN\tLaPorte County\tH1\n46554\t18091\tNorth liberty\tIN\tLaPorte County\tH1\n46383\t18091\tValparaiso\tIN\tLaPorte County\tH1\n46382\t18091\tUnion mills\tIN\tLaPorte County\tH1\n46390\t18091\tWanatah\tIN\tLaPorte County\tH1\n46348\t18091\tLa crosse\tIN\tLaPorte County\tH1\n46371\t18091\tRolling prairie\tIN\tLaPorte County\tH1\n46532\t18091\tHamlet\tIN\tLaPorte County\tH1\n46340\t18091\tHanna\tIN\tLaPorte County\tH1\n46365\t18091\tMill creek\tIN\tLaPorte County\tH1\n46350\t18091\tLa porte\tIN\tLaPorte County\tH1\n46360\t18091\tMichigan city\tIN\tLaPorte County\tH1\n46574\t18091\tWalkerton\tIN\tLaPorte County\tH1\n47108\t18093\tCampbellsburg\tIN\tLawrence County\tH1\n47452\t18093\tOrleans\tIN\tLawrence County\tH1\n47446\t18093\tMitchell\tIN\tLawrence County\tH1\n47420\t18093\tAvoca\tIN\tLawrence County\tH1\n47436\t18093\tHeltonville\tIN\tLawrence County\tH1\n47260\t18093\tMedora\tIN\tLawrence County\tH1\n47462\t18093\tSpringville\tIN\tLawrence County\tH1\n47437\t18093\tHuron\tIN\tLawrence County\tH1\n47421\t18093\tBedford\tIN\tLawrence County\tH1\n47264\t18093\tNorman\tIN\tLawrence County\tH1\n47470\t18093\tWilliams\tIN\tLawrence County\tH1\n47451\t18093\tOolitic\tIN\tLawrence County\tH1\n47467\t18093\tTunnelton\tIN\tLawrence County\tH1\n46040\t18095\tFortville\tIN\tMadison County\tH1\n46012\t18095\tAnderson\tIN\tMadison County\tH1\n46060\t18095\tNoblesville\tIN\tMadison County\tH1\n46056\t18095\tMarkleville\tIN\tMadison County\tH1\n46063\t18095\tOrestes\tIN\tMadison County\tH1\n46013\t18095\tAnderson\tIN\tMadison County\tH1\n46018\t18095\tAnderson\tIN\tMadison County\tH1\n46016\t18095\tAnderson\tIN\tMadison County\tH1\n46011\t18095\tAnderson\tIN\tMadison County\tH1\n46044\t18095\tFrankton\tIN\tMadison County\tH1\n46928\t18095\tFairmount\tIN\tMadison County\tH1\n46001\t18095\tAlexandria\tIN\tMadison County\tH1\n46036\t18095\tElwood\tIN\tMadison County\tH1\n46064\t18095\tPendleton\tIN\tMadison County\tH1\n46048\t18095\tIngalls\tIN\tMadison County\tH1\n46015\t18095\tAnderson\tIN\tMadison County\tH1\n46017\t18095\tAnderson\tIN\tMadison County\tH1\n46070\t18095\tSummitville\tIN\tMadison County\tH1\n47356\t18095\tMiddletown\tIN\tMadison County\tH1\n46051\t18095\tLapel\tIN\tMadison County\tH1\n46201\t18097\tIndianapolis\tIN\tMarion County\tH6\n46268\t18097\tIndianapolis\tIN\tMarion County\tH6\n46226\t18097\tIndianapolis\tIN\tMarion County\tH6\n46229\t18097\tIndianapolis\tIN\tMarion County\tH6\n46204\t18097\tIndianapolis\tIN\tMarion County\tH6\n46244\t18097\tIndianapolis\tIN\tMarion County\tH6\n46230\t18097\tIndianapolis\tIN\tMarion County\tH6\n46249\t18097\tIndianapolis\tIN\tMarion County\tH6\n46203\t18097\tIndianapolis\tIN\tMarion County\tH6\n46260\t18097\tIndianapolis\tIN\tMarion County\tH6\n46280\t18097\tIndianapolis\tIN\tMarion County\tH6\n46290\t18097\tIndianapolis\tIN\tMarion County\tH6\n46222\t18097\tIndianapolis\tIN\tMarion County\tH6\n46221\t18097\tIndianapolis\tIN\tMarion County\tH6\n46228\t18097\tIndianapolis\tIN\tMarion County\tH6\n46250\t18097\tIndianapolis\tIN\tMarion County\tH6\n46037\t18097\tFishers\tIN\tMarion County\tH6\n46183\t18097\tWest newton\tIN\tMarion County\tH6\n46202\t18097\tIndianapolis\tIN\tMarion County\tH6\n46256\t18097\tIndianapolis\tIN\tMarion County\tH6\n46234\t18097\tIndianapolis\tIN\tMarion County\tH6\n46231\t18097\tIndianapolis\tIN\tMarion County\tH6\n46235\t18097\tIndianapolis\tIN\tMarion County\tH6\n46208\t18097\tIndianapolis\tIN\tMarion County\tH6\n46253\t18097\tIndianapolis\tIN\tMarion County\tH6\n46285\t18097\tIndianapolis\tIN\tMarion County\tH6\n46077\t18097\tZionsville\tIN\tMarion County\tH6\n46107\t18097\tBeech grove\tIN\tMarion County\tH6\n46163\t18097\tNew palestine\tIN\tMarion County\tH6\n46113\t18097\tCamby\tIN\tMarion County\tH6\n46278\t18097\tIndianapolis\tIN\tMarion County\tH6\n46225\t18097\tIndianapolis\tIN\tMarion County\tH6\n46236\t18097\tIndianapolis\tIN\tMarion County\tH6\n46237\t18097\tIndianapolis\tIN\tMarion County\tH6\n46242\t18097\tIndianapolis\tIN\tMarion County\tH6\n46241\t18097\tIndianapolis\tIN\tMarion County\tH6\n46240\t18097\tIndianapolis\tIN\tMarion County\tH6\n46283\t18097\tIndianapolis\tIN\tMarion County\tH6\n46298\t18097\tIndianapolis\tIN\tMarion County\tH6\n46254\t18097\tIndianapolis\tIN\tMarion County\tH6\n46220\t18097\tIndianapolis\tIN\tMarion County\tH6\n46217\t18097\tIndianapolis\tIN\tMarion County\tH6\n46224\t18097\tIndianapolis\tIN\tMarion County\tH6\n46219\t18097\tIndianapolis\tIN\tMarion County\tH6\n46206\t18097\tIndianapolis\tIN\tMarion County\tH6\n46247\t18097\tIndianapolis\tIN\tMarion County\tH6\n46227\t18097\tIndianapolis\tIN\tMarion County\tH6\n46251\t18097\tIndianapolis\tIN\tMarion County\tH6\n46259\t18097\tIndianapolis\tIN\tMarion County\tH6\n46216\t18097\tIndianapolis\tIN\tMarion County\tH6\n46218\t18097\tIndianapolis\tIN\tMarion County\tH6\n46205\t18097\tIndianapolis\tIN\tMarion County\tH6\n46239\t18097\tIndianapolis\tIN\tMarion County\tH6\n46214\t18097\tIndianapolis\tIN\tMarion County\tH6\n46282\t18097\tIndianapolis\tIN\tMarion County\tH6\n46213\t18097\tIndianapolis\tIN\tMarion County\tH6\n46504\t18099\tBourbon\tIN\tMarshall County\tH1\n46524\t18099\tEtna green\tIN\tMarshall County\tH1\n46536\t18099\tLakeville\tIN\tMarshall County\tH1\n46570\t18099\tTippecanoe\tIN\tMarshall County\tH1\n46550\t18099\tNappanee\tIN\tMarshall County\tH1\n46563\t18099\tPlymouth\tIN\tMarshall County\tH1\n46506\t18099\tBremen\tIN\tMarshall County\tH1\n46539\t18099\tMentone\tIN\tMarshall County\tH1\n46572\t18099\tTyner\tIN\tMarshall County\tH1\n46537\t18099\tLapaz\tIN\tMarshall County\tH1\n46531\t18099\tGrovertown\tIN\tMarshall County\tH1\n46501\t18099\tArgos\tIN\tMarshall County\tH1\n46574\t18099\tWalkerton\tIN\tMarshall County\tH1\n46511\t18099\tCulver\tIN\tMarshall County\tH1\n46975\t18099\tRochester\tIN\tMarshall County\tH1\n46513\t18099\tDonaldson\tIN\tMarshall County\tH1\n47633\t18101\tPoseyville\tIN\tMartin County\tH1\n47522\t18101\tCrane\tIN\tMartin County\tH1\n47446\t18101\tMitchell\tIN\tMartin County\tH1\n47553\t18101\tLoogootee\tIN\tMartin County\tH1\n47562\t18101\tOdon\tIN\tMartin County\tH1\n47581\t18101\tShoals\tIN\tMartin County\tH1\n47470\t18101\tWilliams\tIN\tMartin County\tH1\n47432\t18101\tFrench lick\tIN\tMartin County\tH1\n47449\t18101\tNewberry\tIN\tMartin County\tH1\n46910\t18103\tAkron\tIN\tMiami County\tH1\n46919\t18103\tConverse\tIN\tMiami County\tH1\n46998\t18103\tYoung america\tIN\tMiami County\tH1\n46958\t18103\tMexico\tIN\tMiami County\tH1\n46959\t18103\tMiami\tIN\tMiami County\tH1\n46974\t18103\tRoann\tIN\tMiami County\tH1\n46936\t18103\tGreentown\tIN\tMiami County\tH1\n46926\t18103\tDenver\tIN\tMiami County\tH1\n46951\t18103\tMacy\tIN\tMiami County\tH1\n46982\t18103\tSilver lake\tIN\tMiami County\tH1\n46921\t18103\tDeedsville\tIN\tMiami County\tH1\n46971\t18103\tGrissom arb\tIN\tMiami County\tH1\n46992\t18103\tWabash\tIN\tMiami County\tH1\n46932\t18103\tGalveston\tIN\tMiami County\tH1\n46901\t18103\tKokomo\tIN\tMiami County\tH1\n46970\t18103\tPeru\tIN\tMiami County\tH1\n46975\t18103\tRochester\tIN\tMiami County\tH1\n46914\t18103\tBunker hill\tIN\tMiami County\tH1\n46911\t18103\tAmboy\tIN\tMiami County\tH1\n47408\t18105\tBloomington\tIN\tMonroe County\tH1\n47433\t18105\tGosport\tIN\tMonroe County\tH1\n47448\t18105\tNashville\tIN\tMonroe County\tH1\n47429\t18105\tEllettsville\tIN\tMonroe County\tH1\n47407\t18105\tBloomington\tIN\tMonroe County\tH1\n47405\t18105\tBloomington\tIN\tMonroe County\tH1\n47464\t18105\tStinesville\tIN\tMonroe County\tH1\n47406\t18105\tBloomington\tIN\tMonroe County\tH1\n47436\t18105\tHeltonville\tIN\tMonroe County\tH1\n47468\t18105\tUnionville\tIN\tMonroe County\tH1\n47401\t18105\tBloomington\tIN\tMonroe County\tH1\n47403\t18105\tBloomington\tIN\tMonroe County\tH1\n47404\t18105\tBloomington\tIN\tMonroe County\tH1\n47462\t18105\tSpringville\tIN\tMonroe County\tH1\n47421\t18105\tBedford\tIN\tMonroe County\t
